vi "S2C_PCIe7841_Proc_DigitalReadRemote.vi"(8 "Error In":errorcluster, 11 "Data":string) -> (0 "Error Out":errorcluster, 3 "State":string)   [LabVIEW 2015]
uses:
  S2C_PCIe7841_Proc_Globals.vi
  <vilib>/Utility/error.llb/Error Cluster From Error Code.vi
  <vilib>/rvi/errors/niLvFpgaAdjustHostInterfaceError.vi
  <vilib>/rvi/interface/nirviReadWriteControl/nirviReadWriteControl.xnode
  NiFpgaLv.dll
  <vilib>/rvi/interface/Simulation/niFpgaSimulationCallBeginRW.vi
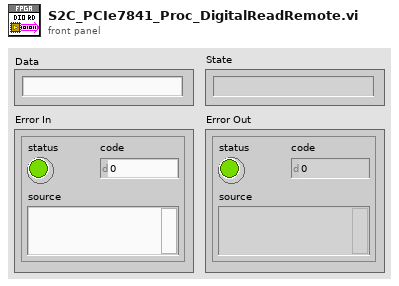
[diagram p1: front panel]
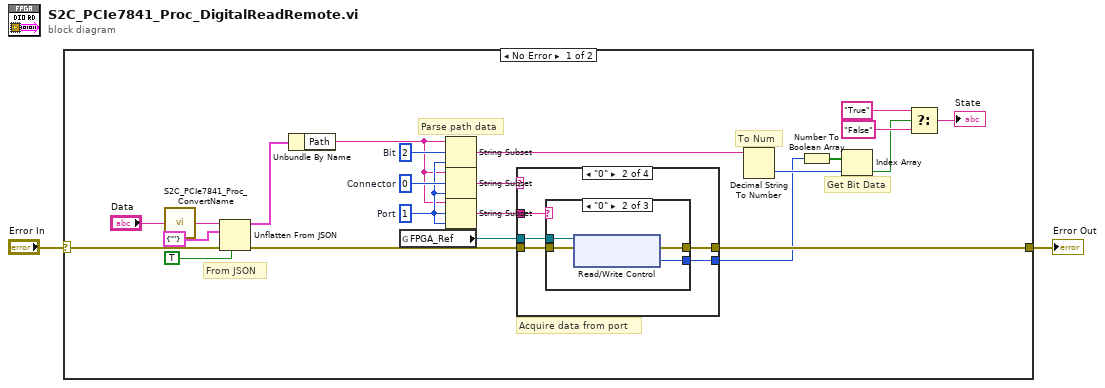
[diagram p0: block diagram]
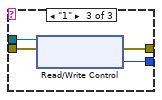
[diagram p4: hidden frame]
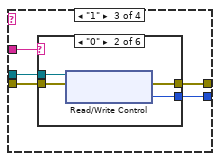
[diagram p5: hidden frame]
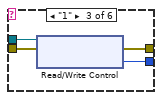
[diagram p7: hidden frame]
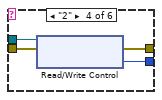
[diagram p8: hidden frame]
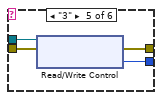
[diagram p9: hidden frame]
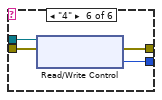
[diagram p10: hidden frame]
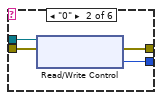
[diagram p12: hidden frame]
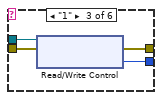
[diagram p13: hidden frame]
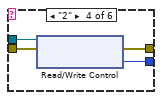
[diagram p14: hidden frame]
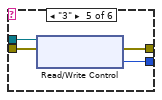
[diagram p15: hidden frame]
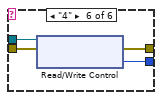
[diagram p16: hidden frame]
diagram:
  n1 = case shown="No Error" "Error In" {
    selector: "Error In" -> [w25 w93]
    tunnel: [w20 w93] -> w1
    frame No Error {
      w7 = 1  # Port
      w8 = 0  # Connector
      w9 = 2  # Bit
      # "Get Bit Data"
      # "Acquire data from port"
      # "Parse path data"
      # "To Num"
      # "From JSON"
      n2 = call "S2C_PCIe7841_Proc_ConvertName.vi"("Data In"="Data") -> ("Data Out"=w10:string)  [unwired: 4 in]
      n3 = Unflatten From JSON(JSON string=w10, type and defaults=cluster{"Path":string} {"Path"=""}, default null elements? (F)=TRUE, error in (no error)=w25) -> (value=w23:cluster{"Path":string}, error out=w21:errorcluster)  [unwired: 3 in]
      n4 = Unbundle By Name(w23) -> ("Path"=w6:string)
      n5 = global read "S2C_PCIe7841_Proc_Globals.vi" "FPGA_Ref"() -> (w12:refnum<k20>)
      n6 = String Subset(string=w6, offset (0)=w9, length (rest)=w7) -> (substring=w3:string)
      n7 = String Subset(string=w6, offset (0)=w8, length (rest)=w7) -> (substring=w5:string)
      n8 = String Subset(string=w6, offset (0)=w7, length (rest)=w7) -> (substring=w4:string)
      n9 = case shown="\"0\"" w5 {
        tunnel: w21 -> [w26 w31 w45 w71]
        tunnel: [w26 w30 w44 w70] -> w20
        tunnel: [_ w29 w43 w69] -> w17
        tunnel: w12 -> [_ w28 w42 w68]
        tunnel: w4 -> [_ w27 w41 w67]
        frame "4", Default {
        }
        frame "0" {
          n10 = case shown="\"0\"" w27 {
            tunnel: w31 -> [w32 w36 w40]
            tunnel: [w32 w35 w39] -> w30
            tunnel: [_ w34 w38] -> w29
            tunnel: w28 -> [_ w33 w37]
            frame "5", Default {
            }
            frame "0" {
              n11 = xnode "Read/Write Control"("FPGA VI Reference In"=w33, "error in"=w36) -> ("error out"=w35:errorcluster, "Conn0/Port0"=w34:u8)  [unwired: 1 out]
            }
            frame "1" {
              n12 = xnode "Read/Write Control"("FPGA VI Reference In"=w37, "error in"=w40) -> ("error out"=w39:errorcluster, "Conn0/Port1"=w38:u8)  [unwired: 1 out]
            }
          }
        }
        frame "1" {
          n13 = case shown="\"0\"" w41 {
            tunnel: w45 -> [w46 w50 w54 w58 w62 w66]
            tunnel: [w46 w49 w53 w57 w61 w65] -> w44
            tunnel: [_ w48 w52 w56 w60 w64] -> w43
            tunnel: w42 -> [_ w47 w51 w55 w59 w63]
            frame "5", Default {
            }
            frame "0" {
              n14 = xnode "Read/Write Control"("FPGA VI Reference In"=w47, "error in"=w50) -> ("error out"=w49:errorcluster, "Conn1/Port0"=w48:u8)  [unwired: 1 out]
            }
            frame "1" {
              n15 = xnode "Read/Write Control"("FPGA VI Reference In"=w51, "error in"=w54) -> ("error out"=w53:errorcluster, "Conn1/Port1"=w52:u8)  [unwired: 1 out]
            }
            frame "2" {
              n16 = xnode "Read/Write Control"("FPGA VI Reference In"=w55, "error in"=w58) -> ("error out"=w57:errorcluster, "Conn1/Port2"=w56:u8)  [unwired: 1 out]
            }
            frame "3" {
              n17 = xnode "Read/Write Control"("FPGA VI Reference In"=w59, "error in"=w62) -> ("error out"=w61:errorcluster, "Conn1/Port3"=w60:u8)  [unwired: 1 out]
            }
            frame "4" {
              n18 = xnode "Read/Write Control"("FPGA VI Reference In"=w63, "error in"=w66) -> ("error out"=w65:errorcluster, "Conn1/Port4"=w64:u8)  [unwired: 1 out]
            }
          }
        }
        frame "2" {
          n19 = case shown="\"5\", Default" w67 {
            tunnel: w71 -> [w72 w76 w80 w84 w88 w92]
            tunnel: [w72 w75 w79 w83 w87 w91] -> w70
            tunnel: [_ w74 w78 w82 w86 w90] -> w69
            tunnel: w68 -> [_ w73 w77 w81 w85 w89]
            frame "5", Default {
            }
            frame "0" {
              n20 = xnode "Read/Write Control"("FPGA VI Reference In"=w73, "error in"=w76) -> ("error out"=w75:errorcluster, "Conn2/Port0"=w74:u8)  [unwired: 1 out]
            }
            frame "1" {
              n21 = xnode "Read/Write Control"("FPGA VI Reference In"=w77, "error in"=w80) -> ("error out"=w79:errorcluster, "Conn2/Port1"=w78:u8)  [unwired: 1 out]
            }
            frame "2" {
              n22 = xnode "Read/Write Control"("FPGA VI Reference In"=w81, "error in"=w84) -> ("error out"=w83:errorcluster, "Conn2/Port2"=w82:u8)  [unwired: 1 out]
            }
            frame "3" {
              n23 = xnode "Read/Write Control"("FPGA VI Reference In"=w85, "error in"=w88) -> ("error out"=w87:errorcluster, "Conn2/Port3"=w86:u8)  [unwired: 1 out]
            }
            frame "4" {
              n24 = xnode "Read/Write Control"("FPGA VI Reference In"=w89, "error in"=w92) -> ("error out"=w91:errorcluster, "Conn2/Port4"=w90:u8)  [unwired: 1 out]
            }
          }
        }
      }
      n25 = Decimal String To Number(string=w3) -> (number=w19:i32)  [unwired: 2 in, 1 out]
      n26 = Number To Boolean Array(number=w17) -> (Boolean array=w18:bool[])
      n27 = Index Array(array=w18, index=w19) -> (element=w14:bool)
      n28 = Select(t="True", s=w14, f="False") -> (s? t:f=→"State":string)
    }
    frame Error {
    }
  }
  "Error Out" <- w1
